vi "Initialize.vi"(9 "result":bool, 10 "time/date":timestamp=timestamp(3230114789.968 s since 1904-01-01)) -> (3 "Test Results":refnum<class "Test Results Base Class.lvclass">)   [LabVIEW 2020, in "Test Results Base Class.lvclass"]
doc: "This VI initializes the data members of the class \"Test Results Parent Class.\""
uses:
  Test Results Base Class.lvclass
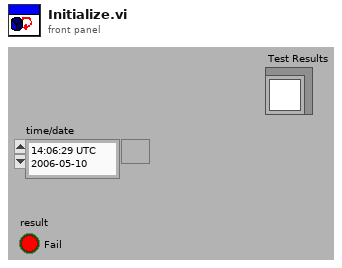
[diagram p1: front panel]
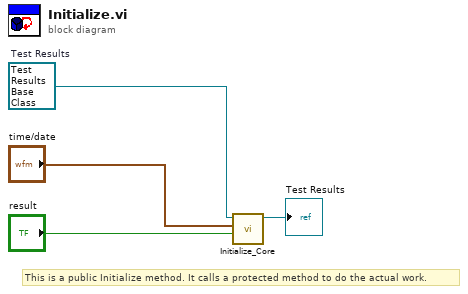
[diagram p0: block diagram]
diagram:
  w4 = refnum<class "Test Results Base Class.lvclass"> refnum  # Test Results
  # "This is a public Initialize method. It calls a protected method to do the actual work."
  n1 = call "Initialize_Core.vi"("result"="result", "time/date"="time/date", "Test Results \nParent Class in"=w4) -> ("Test Results\nParent Class out"=→"Test Results":refnum<class "Test Results Base Class.lvclass">)  [unwired: 8 in]
